vi "Labview Project Credits .vi"() -> ()   [LabVIEW 2025]
panel:
  out "Message":string
  in  "Credits":i32
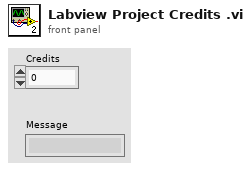
[diagram p1: front panel]
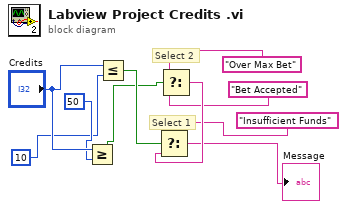
[diagram p0: block diagram]
diagram:
  # "Select 2"
  # "Select 1"
  n1 = Greater Or Equal?(x="Credits", y=50) -> (x >= y?=w3:bool)
  n2 = Less Or Equal?(x="Credits", y=10) -> (x <= y?=w4:bool)
  n3 = Select(t="Over Max Bet", s=w3, f="Bet Accepted") -> (s? t:f=w9:string)
  n4 = Select(t="Insufficient Funds", s=w4, f=w9) -> (s? t:f=→"Message":string)
